vi "Read New Transaction.vi"(8 "error in (no error)":errorcluster, 9 "State":T1=enum."Terminate", 10 "Target time":dbl=10.0 format="%#_13g", 11 "Sim User Console Actor in":refnum<class "Sim User Console Actor.lvclass">) -> (0 "error out":errorcluster, 3 "Sim User Console Actor out":refnum<class "Sim User Console Actor.lvclass">)   [LabVIEW 2019, in "Sim User Console Actor.lvlib" / "Sim User Console Actor.lvclass"]
uses:
  Sim User Console Actor.lvclass
  C:/Program Files (x86)/National Instruments/LabVIEW 2019/vi.lib/ActorFramework/Actor/Actor.lvclass
  ATM Controller/ATM Controller/State -Enum.ctl
  <vilib>/ActorFramework/Actor/Actor.lvclass/Actor.ctl
  Sim User Console Actor.lvclass/Sim User Console Actor.ctl
  ATM Controller/ATM Controller Messages/Set Timer Msg/Set Timer Msg.lvclass/Set Timer Msg.ctl
  <vilib>/ActorFramework/Message Enqueuer/Message Enqueuer.lvclass/Message Enqueuer.ctl
  <vilib>/ActorFramework/Message Enqueuer/Enqueue.vi
  ATM Controller/ATM Controller Messages/Set Timer Msg/Set Timer Msg.lvclass
  C:/Program Files (x86)/National Instruments/LabVIEW 2019/vi.lib/ActorFramework/Message/Message.lvclass
  <vilib>/ActorFramework/Message Priority Queue/Priority Enqueue.vi
  <vilib>/ActorFramework/Actor/Actor.lvclass
  ATM Controller/ATM Controller/ATM Controller.lvclass
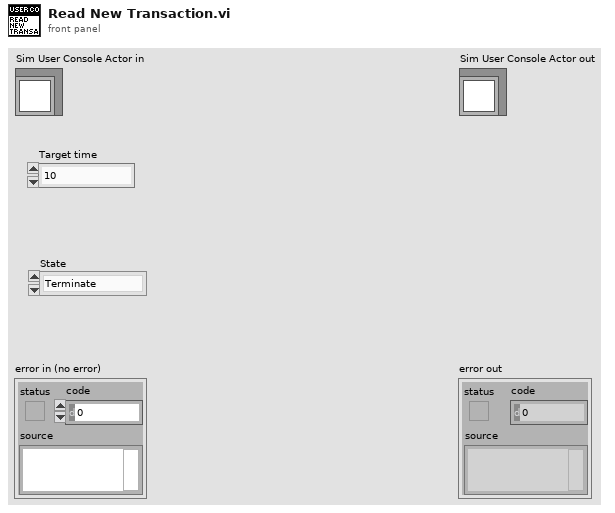
[diagram p1: front panel]
types:
  T1 = typedef "ATM Controller.lvlib/ATM Controller.lvclass/State -Enum.ctl" = enum16{"Initial", "Idle", "Login", "Balance Inquiry", "Deposit", "Withdrawal", "Fast Cash", "Terminate", "Inactivity Timeout"}
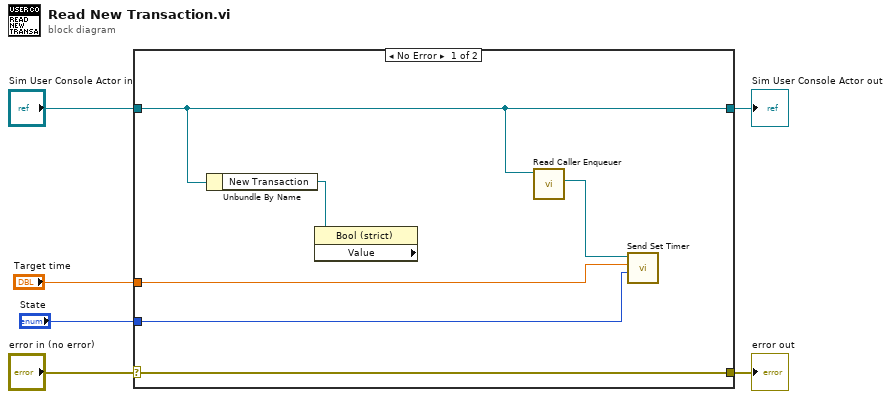
[diagram p0: block diagram]
diagram:
  n1 = case shown="No Error" "error in (no error)" {
    selector: "error in (no error)" -> [w12 w14]
    tunnel: [w12 w14] -> w5
    tunnel: [w9 w13] -> w3
    tunnel: "Sim User Console Actor in" -> [w9 w13]
    tunnel: "Target time" -> [w8 _]
    tunnel: "State" -> [w7 _]
    frame No Error {
      n2 = Unbundle By Name(w9) -> ("New Transaction"=w10:refnum<vi>)
      n3 = property class="Bool (strict)" props=["Value"](reference=w10) -> ()  [unwired: 1 in, 3 out]
      n4 = call <vilib>:"Read Caller Enqueuer.vi"("Actor"=w9) -> ("Caller Enqueuer"=w11:refnum<class "Message Enqueuer.lvclass">)  [unwired: 10 in]
      n5 = call "Send Set Timer.vi"("State"=w7, "Target time"=w8, "Message Enqueuer"=w11) -> ()  [unwired: 7 in, 2 out]
    }
    frame Error {
    }
  }
  "error out" <- w5
  "Sim User Console Actor out" <- w3
